vi "Self-Test.vi"(8 "error in (no error)":errorcluster, 11 "VISA resource name":refnum<visa-resource-name>) -> (0 "error out":errorcluster, 1 "Self Test successful":bool, 2 "Self-Test Result Code":i32, 3 "VISA resource name out":refnum<visa-resource-name>, 4 "Device Errors":cluster{"code":i32, "Text":string}[](array[cluster]))   [LabVIEW 2014, in "Stanford Research DG645 - Driver.lvlib"]
doc: "Common IEEE-488.2 Command: *TST?\nInstrument Error Check\n\nRuns the instrument self test and returns 0 if successful and 16 if unsuccessful. If unsuccessful the error buffer will include device dependent errors related to the parts of the self test that failed."
uses:
  Stanford Research DG645 - Driver.lvlib
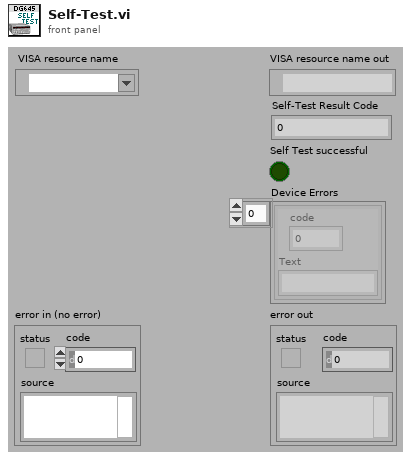
[diagram p1: front panel]
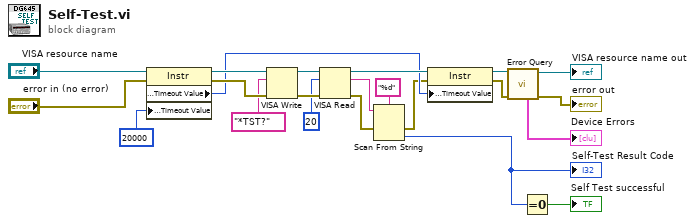
[diagram p0: block diagram]
diagram:
  n1 = property class="Instr"(reference="VISA resource name", error in="error in (no error)", "General Settings:Timeout Value"=u32 20000 ("Timeout")) -> (reference out=w10:refnum<visa-resource-name>, error out=w11:errorcluster, "General Settings:Timeout Value"=w9:u32)
  n2 = VISA Write(VISA resource name=w10, write buffer="*TST?" ("Self-Test Command"), error in (no error)=w11) -> (VISA resource name out=w20:refnum<visa-resource-name>, error out=w19:errorcluster)  [unwired: 1 out]
  n3 = VISA Read(VISA resource name=w20, byte count=u32 20 ("byte count (20)"), error in (no error)=w19) -> (VISA resource name out=w21:refnum<visa-resource-name>, read buffer=w15:string, error out=w2:errorcluster)  [unwired: 1 out]
  n4 = Scan From String(format string="%d", input string=w15, error in=w2) -> (error out=w1:errorcluster, output 1=w5:i32)  [unwired: 2 in, 2 out]
  "Self-Test Result Code" <- w5
  n5 = property class="Instr"(reference=w21, error in=w1, "General Settings:Timeout Value"=w9) -> (reference out=w3:refnum<visa-resource-name>, error out=w4:errorcluster)
  n6 = call "Error Query.vi"("error in (no error)"=w4, "VISA resource name"=w3) -> ("error out"=→"error out":errorcluster, "VISA resource name out"=→"VISA resource name out":refnum<visa-resource-name>, "Device Errors"=→"Device Errors":cluster{"code":i32, "Text":string}[])  [unwired: 7 in]
  n7 = Equal To 0?(x=w5) -> (x = 0?=→"Self Test successful":bool)
